vi "Get Wire Class Query terms.vi"(1 "App Refnum":refnum<vi>, 2 "Project Item Names":string[](array[string])=["Parrent.lvclass [My Computer< Untitled Project 1.lvproj]", "Child.lvclass [My Computer< Untitled Project 1.lvproj]", "QD Test.vi [My Computer< Untitled Project 1.lvproj]", "Find Project Items.vi [QuickDrop< My Computer< Untitled Project 1.lvproj]", "Get Default QD Object Shortcuts File.vi [QuickDrop< My Computer< Untitled Project 1.lvproj]", "Load Default QD Object Shortcuts.vi [QuickDrop< My Computer< Untitled Project 1.lvproj]", "OldSearchAlgorithm.vi [QuickDrop< My Computer< Untitled Project 1.lvproj]", "OpenSearchWrapper.vi [QuickDrop< My Computer< Untitled Project 1.lvproj]", "QuickDrop Get QDKS Info for Shortcut Dialog.vi [QuickDrop< My Computer< Untitled Project 1.lvproj]", "QuickDrop Get QDKS Mappings.vi [QuickDrop< My Computer< Untitled Project 1.lvproj]", "QuickDrop Get Shortcut Info.vi [QuickDrop< My Computer< Untitled Project 1.lvproj]", "QuickDrop Get Terminal Names.vi [QuickDrop< My Computer< Untitled Project 1.lvproj]", "QuickDrop Get Wire Prefix.vi [QuickDrop< My Computer< Untitled Project 1.lvproj]", "QuickDrop Launch Window.vi [QuickDrop< My Computer< Untitled Project 1.lvproj]", "QuickDrop Get Wire Query terms.vi [QuickDrop< My Computer< Untitled Project 1.lvproj]", "QuickDrop Insert String into Array.vi [QuickDrop< My Computer< Untitled Project 1.lvproj]", "QuickDrop Plugin Template.vit [QuickDrop< My Computer< Untitled Project 1.lvproj]", "QuickDrop Populate QDKS Listbox.vi [QuickDrop< My Computer< Untitled Project 1.lvproj]", "QuickDrop Process Drop Information.vi [QuickDrop< My Computer< Untitled Project 1.lvproj]", "QuickDrop QDKS Info.ctl [QuickDrop< My Computer< Untitled Project 1.lvproj]", "QuickDrop Read QDKS INI Info.vi [QuickDrop< My Computer< Untitled Project 1.lvproj]", "QuickDrop Shortcut Config.vi [QuickDrop< My Computer< Untitled Project 1.lvproj]", "QuickDrop Get Wire Class Query terms.vi [QuickDrop< My Computer< Untitled Project 1.lvproj]", "Parrent_Create.vi [Parrent.lvclass< My Computer< Untitled Project 1.lvproj]", "Destroy.vi [Parrent.lvclass< My Computer< Untitled Project 1.lvproj]", "Child_Create.vi [Child.lvclass< My Computer< Untitled Project 1.lvproj]", "Destroy.vi [Child.lvclass< My Computer< Untitled Project 1.lvproj]", "Method 1.vi [Child.lvclass< My Computer< Untitled Project 1.lvproj]", "Method 2.vi [Child.lvclass< My Computer< Untitled Project 1.lvproj]", "LV Config Read.vi [Dependencies< My Computer< Untitled Project 1.lvproj]", "LV Config Read Boolean.vi [Dependencies< My Computer< Untitled Project 1.lvproj]", "LV Config Read String.vi [Dependencies< My Computer< Untitled Project 1.lvproj]", "LV Config Read Pathlist.vi [Dependencies< My Computer< Untitled Project 1.lvproj]", "LV Config Read Color.vi [Dependencies< My Computer< Untitled Project 1.lvproj]", "LV Config Read Numeric (I32).vi [Dependencies< My Computer< Untitled Project 1.lvproj]", "LV Config Write.vi [Dependencies< My Computer< Untitled Project 1.lvproj]", "LV Config Write Boolean.vi [Dependencies< My Computer< Untitled Project 1.lvproj]", "LV Config Write String.vi [Dependencies< My Computer< Untitled Project 1.lvproj]", "LV Config Write Pathlist.vi [Dependencies< My Computer< Untitled Project 1.lvproj]", "LV Config Write Color.vi [Dependencies< My Computer< Untitled Project 1.lvproj]", "LV Config Write Numeric (I32).vi [Dependencies< My Computer< Untitled Project 1.lvproj]", "VSI TSVN Tbar_SVN Lock with Dialog.vi [Dependencies< My Computer< Untitled Project 1.lvproj]", "VSI TSVN Tbar_Handle SVN Error.vi [Dependencies< My Computer< Untitled Project 1.lvproj]", "Status Dialog Display Button.vi [Dependencies< My Computer< Untitled Project 1.lvproj]", "Status Dialog Justify Text.vi [Dependencies< My Computer< Untitled Project 1.lvproj]", "Status Dialog Update Message.vi [Dependencies< My Computer< Untitled Project 1.lvproj]", "Status Dialog Exit.vi [Dependencies< My Computer< Untitled Project 1.lvproj]", "Status Dialog Init.vi [Dependencies< My Computer< Untitled Project 1.lvproj]", "Status Dialog Wait for Status Queue.vi [Dependencies< My Computer< Untitled Project 1.lvproj]", "Status Dialog.vi [Dependencies< My Computer< Untitled Project 1.lvproj]", "Insert.vi [plugins< QuickDrop< My Computer< Untitled Project 1.lvproj]", "Move Labels.vi [plugins< QuickDrop< My Computer< Untitled Project 1.lvproj]", "Remove and Rewire.vi [plugins< QuickDrop< My Computer< Untitled Project 1.lvproj]", "Replace.vi [plugins< QuickDrop< My Computer< Untitled Project 1.lvproj]", "SVN Commit.vi [plugins< QuickDrop< My Computer< Untitled Project 1.lvproj]", "SVN Lock.vi [plugins< QuickDrop< My Computer< Untitled Project 1.lvproj]", "SVN Update.vi [plugins< QuickDrop< My Computer< Untitled Project 1.lvproj]", "VI Server Rename.vi [plugins< QuickDrop< My Computer< Untitled Project 1.lvproj]", "Wire All Terminals.vi [plugins< QuickDrop< My Computer< Untitled Project 1.lvproj]", "Wire Multiple Objects Together.vi [plugins< QuickDrop< My Computer< Untitled Project 1.lvproj]", "ObjectAttributes.ctl [protected< Parrent.lvclass< My Computer< Untitled Project 1.lvproj]", "Parrent_New.vi [utils< Parrent.lvclass< My Computer< Untitled Project 1.lvproj]", "Parrent_GetAttributes.vi [utils< Parrent.lvclass< My Computer< Untitled Project 1.lvproj]", "ObjectAttributes.ctl [protected< Child.lvclass< My Computer< Untitled Project 1.lvproj]", "Child_New.vi [utils< Child.lvclass< My Computer< Untitled Project 1.lvproj]", "Child_GetAttributes.vi [utils< Child.lvclass< My Computer< Untitled Project 1.lvproj]", "TTK_FTW-ERR-CallChain.vi [TTK_FTW.lvlib< Dependencies< My Computer< Untitled Project 1.lvproj]", "TTK_FTW-ERR-Clear.vi [TTK_FTW.lvlib< Dependencies< My Computer< Untitled Project 1.lvproj]", "TTK_FTW-ERR-NoErrorConstant.vi [TTK_FTW.lvlib< Dependencies< My Computer< Untitled Project 1.lvproj]", "TTK_FTW-ERR-ThrowError.vi [TTK_FTW.lvlib< Dependencies< My Computer< Untitled Project 1.lvproj]", "TTK_FTW-Regex-ReplaceAll.vi [TTK_FTW.lvlib< Dependencies< My Computer< Untitled Project 1.lvproj]", "TTK_FTW-Regex.vi [TTK_FTW.lvlib< Dependencies< My Computer< Untitled Project 1.lvproj]", "TTK_FTW-STR-Array-Delimit.vi [TTK_FTW.lvlib< Dependencies< My Computer< Untitled Project 1.lvproj]", "TTK_FTW-STR-ReplaceWhitespace.vi [TTK_FTW.lvlib< Dependencies< My Computer< Untitled Project 1.lvproj]", "Available Non-Node.ctl [_WireMultipleSupport< plugins< QuickDrop< My Computer< Untitled Project 1.lvproj]", "Change Tunnel Modes to Fix Wires.vi [_WireMultipleSupport< plugins< QuickDrop< My Computer< Untitled Project 1.lvproj]", "Connect Valid Terminals.vi [_WireMultipleSupport< plugins< QuickDrop< My Computer< Untitled Project 1.lvproj]", "Connector Pane Position.ctl [_WireMultipleSupport< plugins< QuickDrop< My Computer< Untitled Project 1.lvproj]", "Find Top and Error Terminals.vi [_WireMultipleSupport< plugins< QuickDrop< My Computer< Untitled Project 1.lvproj]", "Get Wirable Objects from Selection.vi [_WireMultipleSupport< plugins< QuickDrop< My Computer< Untitled Project 1.lvproj]", "Group Selection List By Row.vi [_WireMultipleSupport< plugins< QuickDrop< My Computer< Untitled Project 1.lvproj]", "Match Relaxed Data Type.vi [_WireMultipleSupport< plugins< QuickDrop< My Computer< Untitled Project 1.lvproj]", "Match Source and Sink Terminals.vi [_WireMultipleSupport< plugins< QuickDrop< My Computer< Untitled Project 1.lvproj]", "Node Terminal Info.ctl [_WireMultipleSupport< plugins< QuickDrop< My Computer< Untitled Project 1.lvproj]", "Node-Terminal Pair.ctl [_WireMultipleSupport< plugins< QuickDrop< My Computer< Untitled Project 1.lvproj]", "Prepare to Wire Two Nodes.vi [_WireMultipleSupport< plugins< QuickDrop< My Computer< Untitled Project 1.lvproj]", "Sort Node Terminals.vi [_WireMultipleSupport< plugins< QuickDrop< My Computer< Untitled Project 1.lvproj]", "Sort Unwired Terminals.vi [_WireMultipleSupport< plugins< QuickDrop< My Computer< Untitled Project 1.lvproj]", "What to Wire.ctl [_WireMultipleSupport< plugins< QuickDrop< My Computer< Untitled Project 1.lvproj]", "Wire Non-Nodes to Nodes.vi [_WireMultipleSupport< plugins< QuickDrop< My Computer< Untitled Project 1.lvproj]"], 3 "Project Item Refs":refnum<vi>[](array[refnum]), 7 "Class/vi name":string="Child.lvclass", 11 "error in (no error)":errorcluster) -> (4 "Class Item Names":string[](array[string]), 15 "error out":errorcluster)   [LabVIEW 2018]
doc: "Created by VI-Tech"
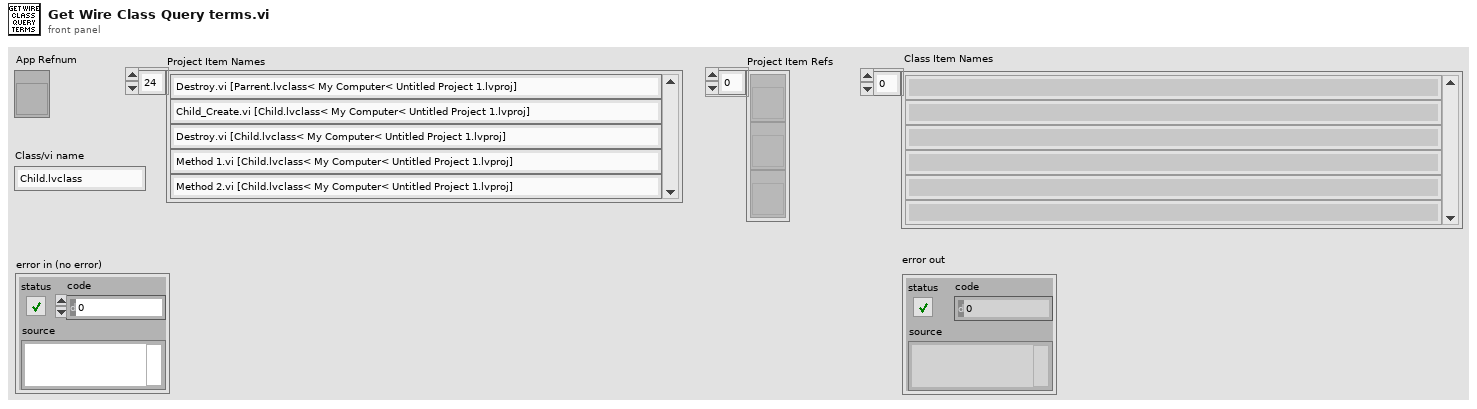
[diagram p1: front panel]
types:
  T1 = enum32{"invalid scope", "public", "private", "protected", "community"}
  T2 = enum32{"invalid scope", "public", "private", "protected", "community"}[]
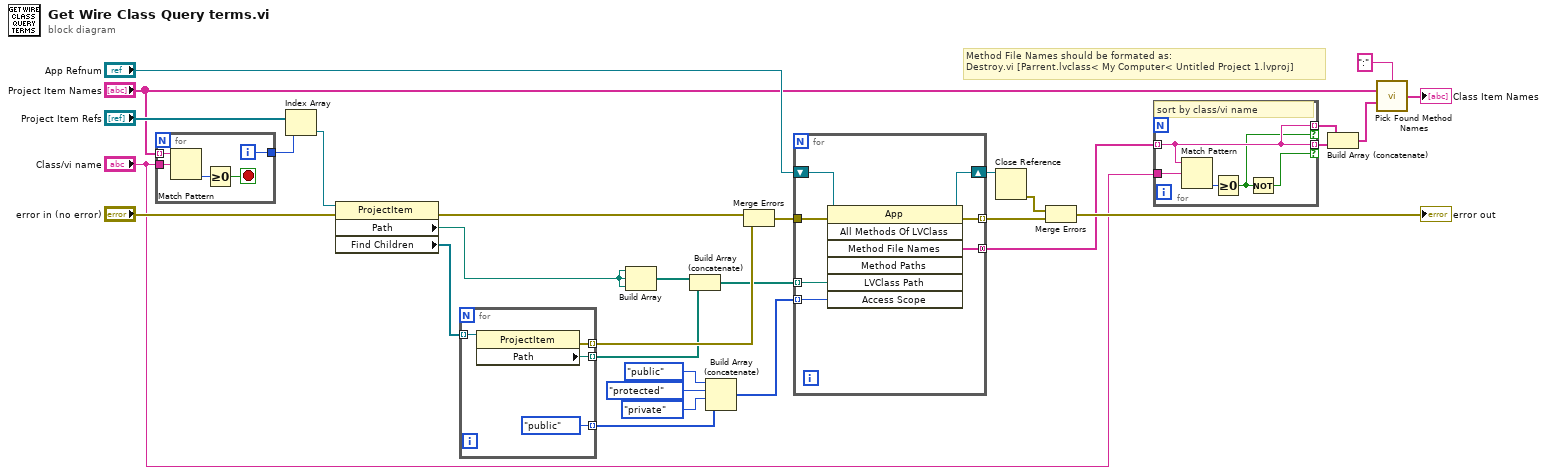
[diagram p0: block diagram]
diagram:
  # "Method File Names should be formated as:\nDestroy.vi [Parrent.lvclass< My Computer< Untitled Project 1.lvproj]"
  n1 = for {
    tunnel: "Project Item Names" -> [w33] mode=indexing
    tunnel: "Class/vi name" -> [w35]
    tunnel: [w31] -> w15
    i -> [w31]
    stop <- w32 stop-if-true
    n2 = Match Pattern(string=w33, regular expression=w35) -> (offset past match=w34:i32)  [unwired: 1 in, 3 out]
    n3 = Greater Or Equal To 0?(x=w34) -> (x >= 0?=w32:bool)
  }
  n4 = Index Array(array="Project Item Refs", index=w15) -> (element=w13:refnum<vi>)
  n5 = property class="ProjectItem"(reference=w13, error in="error in (no error)") -> (error out=w10:errorcluster, "Path"=w12:path, "Find Children"=w14:refnum<vi>[])  [unwired: 1 out]
  n6 = for {
    tunnel: w14 -> [w36] mode=indexing
    tunnel: [w39] -> w26 mode=indexing
    tunnel: [w38] -> w30 mode=indexing
    tunnel: [T1."public" ("Access Scope")] -> w19 mode=indexing
    n7 = property class="ProjectItem"(reference=w36) -> (error out=w38:errorcluster, "Path"=w39:path)  [unwired: 1 in, 1 out]
  }
  n8 = Build Array(w12, w12, w12) -> (w23:path[])
  n9 = Build Array (concatenate)(w23, w26) -> (w11:path[])
  n10 = Build Array (concatenate)(T1."public" ("Access Scope"), T1."protected" ("Access Scope"), T1."private" ("Access Scope"), w19) -> (w18:T2)
  n11 = Merge Errors(w10, w30) -> (w25:errorcluster)
  n12 = for {
    tunnel: w25 -> [w46]
    tunnel: w11 -> [w45] mode=indexing
    tunnel: [w44] -> w24 mode=indexing
    tunnel: w18 -> [w42] mode=indexing
    shift-right: [w41] -> w17
    shift-left: "App Refnum" -> [w43]
    tunnel: [w40] -> w5 mode=concatenating
    n13 = invoke class="App" method="All Methods Of LVClass"(reference=w43, error in=w46, "LVClass Path"=w45, "Access Scope"=w42) -> (reference out=w41:refnum<vi>, error out=w44:errorcluster, "Method File Names"=w40:string[])  [unwired: 3 in, 4 out]
  }
  n14 = Close Reference(reference=w17) -> (error out=w16:errorcluster)  [unwired: 1 in]
  n15 = Merge Errors(w16, w24) -> (→"error out":errorcluster)
  n16 = for {
    tunnel: w5 -> [w50] mode=indexing
    tunnel: "Class/vi name" -> [w51]
    tunnel: [w50] -> w2 mode=indexing if=w48
    tunnel: [w50] -> w3 mode=indexing if=w49
    # "sort by class/vi name"
    n17 = Match Pattern(string=w50, regular expression=w51) -> (offset past match=w47:i32)  [unwired: 1 in, 3 out]
    n18 = Greater Or Equal To 0?(x=w47) -> (x >= 0?=w49:bool)
    n19 = Not(x=w49) -> (.not. x?=w48:bool)
  }
  n20 = Build Array (concatenate)(w3, w2) -> (w1:string[])
  n21 = call "Pick Found Method Names.vi"("delimiter"=":", "Project Item Names"="Project Item Names", "Method File Names"=w1) -> ("Method File Names"=→"Class Item Names":string[])  [unwired: 12 in]
